vi "DVR Creator.vi"() -> ()   [LabVIEW 2023]
doc: "This Vi acts as a DVR creater where a Data Value Reference is created for the particular data and can be modified by incrementing it."
uses:
  Controls/StoreRef.ctl
panel:
  out "error out":errorcluster
  in  "error in (no error)":errorcluster
  in  "Increment":bool
  in  "Stop":bool
  in  "Data":dbl
  # "Instructions:\n\n-> Run the Vi.\n-> Give the input value to data.\n-> Press increment button to increment the value\n-> The incremented output will be displayed in Display Value.vi\n-> Run the Display Value.vi and press Get Value button to see \n     the output value.\n-> Press STOP to stop the running vi."
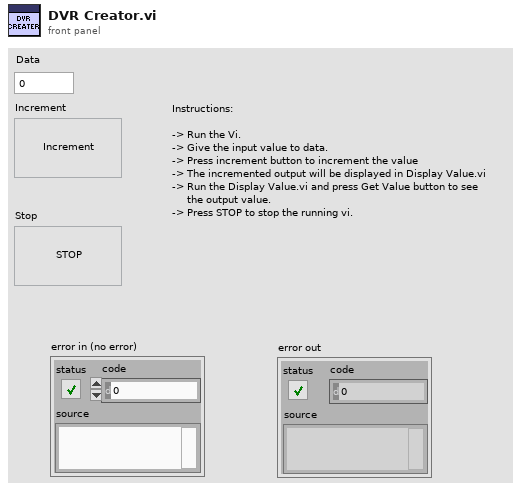
[diagram p1: front panel]
types:
  T1 = typedef "StoreRef.ctl" = enum16{"Store Ref", "Get Ref"}
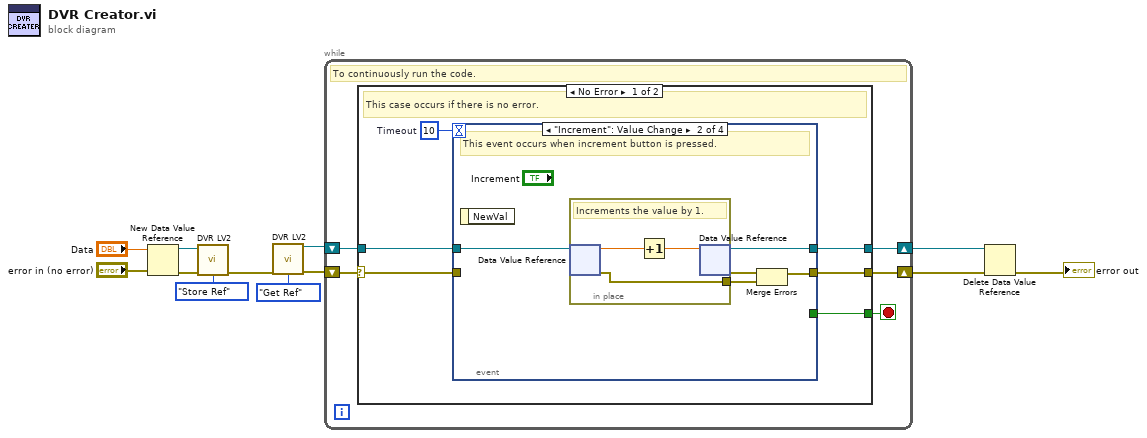
[diagram p0: block diagram]
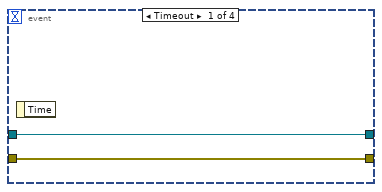
[diagram p2: hidden frame]
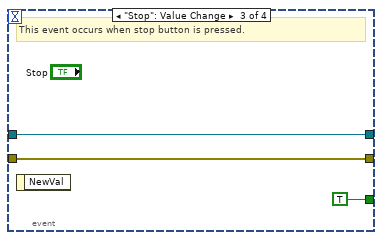
[diagram p3: hidden frame]
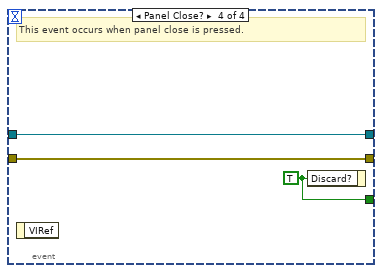
[diagram p4: hidden frame]
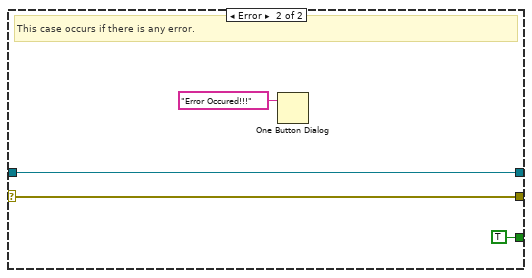
[diagram p5: hidden frame]
diagram:
  n1 = New Data Value Reference(data value="Data", error in="error in (no error)") -> (data value reference=w8:refnum<data-value>, error out=w9:errorcluster)
  n2 = call "DVR LV2.vi"("Data Value Reference"=w8, "error in (no error)"=w9, "Operation"=StoreRef."Store Ref") -> ("error out"=w7:errorcluster)  [unwired: 11 in, 1 out]
  n3 = call "DVR LV2.vi"("error in (no error)"=w7, "Operation"=StoreRef."Get Ref") -> ("Data Value Reference Out"=w6:refnum<data-value>, "error out"=w5:errorcluster)  [unwired: 12 in]
  n4 = while {
    shift-right: [w14] -> w3
    shift-left: w6 -> [w17]
    shift-right: [w15] -> w10
    shift-left: w5 -> [w16]
    stop <- w13 stop-if-true
    # "To continuously run the code."
    n5 = case shown="No Error" w16 {
      selector: w16 -> [w21 w43]
      tunnel: w17 -> [w22 w42]
      tunnel: [w20 w43] -> w15
      tunnel: [w19 w42] -> w14
      tunnel: [w18 TRUE ("Discard?")] -> w13
      frame No Error {
        w23 = 10  # Timeout
        # "This case occurs if there is no error."
        n6 = event shown="[1] \"Increment\": Value Change" {
          selector: _ -> [_ _ _ _]
          dyn-events: _ -> [_ _ _ _]
          timeout: w23 -> [_ _ _ _]
          tunnel: w22 -> [w24 w30 w36 w39]
          tunnel: [w24 w29 w36 w39] -> w19
          tunnel: [w25 w26 w35 w38] -> w20
          tunnel: w21 -> [w25 _ w35 w38]
          tunnel: [_ _ TRUE w37] -> w18
          event Timeout {
            n7 = event-data() -> ()  [unwired: 1 in, 1 out]
          }
          event "Increment": Value Change {
            # "This event occurs when increment button is pressed."
            n8 = event-data() -> ()  [unwired: 1 in, 1 out]
            n9 = in-place {
              in-place-border: [w31] -> w27
              # "Increments the value by 1."
              n10 = in-place-dvr #1(w30) -> (w33:dbl, w31:errorcluster)
              n11 = Increment(x=w33) -> (x+1=w32:dbl)
              n12 = in-place-dvr #1(w32) -> (w29:refnum<data-value>, w28:errorcluster)
            }
            n13 = Merge Errors(w28, w27) -> (w26:errorcluster)
          }
          event "Stop": Value Change {
            # "This event occurs when stop button is pressed."
            n14 = event-data() -> ()  [unwired: 1 in, 1 out]
          }
          event Panel Close? {
            w37 = TRUE ("Discard?")
            # "This event occurs when panel close is pressed."
            n15 = event-data() -> ()  [unwired: 1 in, 1 out]
            n16 = event-data("Discard?"=w37) -> ()  [unwired: 1 in, 1 out]
          }
        }
      }
      frame Error {
        # "This case occurs if there is any error."
        n17 = One Button Dialog(message="Error Occured!!!") -> ()  [unwired: 1 in, 1 out]
      }
    }
  }
  n18 = Delete Data Value Reference(data value reference=w3, error in=w10) -> (error out=→"error out":errorcluster)  [unwired: 1 out]
